vi "获取特殊单位符号字符（菜单下拉列表）.vi"(11 "特殊单位符号":T1 items=["°", "′", "″", "＄", "￥", "〒", "￠", "￡", "％", "＠", "℃", "℉", "﹩", "﹪", "‰", "﹫", "㏕", "㎜", "㎝", "㎞", "㏎", "㎡", "㎎", "㎏", "㏄", "°", "○", "¤", ""]) -> (3 "字符（双字节）":string)   [LabVIEW 2012]
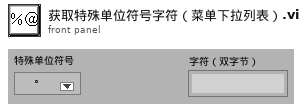
[diagram p1: front panel]
types:
  T1 = typedef "特殊单位符号菜单列表.ctl" = u16
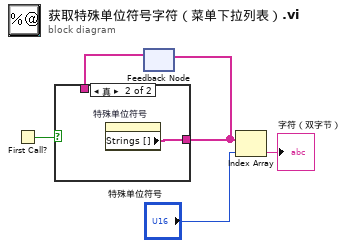
[diagram p0: block diagram]
diagram:
  n1 = First Call?() -> (First Call?: T/F=w5:bool)
  n2 = feedback #1() -> (w3:string[])  [unwired: 1 in]
  n3 = case shown="真" w5 {
    tunnel: [w6 w7] -> w4
    tunnel: w3 -> [w6 _]
    frame False {
    }
    frame True {
      n4 = property on="特殊单位符号" class="Ring (严格)"() -> ("Strings []"=w7:string[])  [unwired: 2 in, 2 out]
    }
  }
  n5 = feedback-in #1(w4) -> ()
  n6 = Index Array(array=w4, index="特殊单位符号") -> (element=→"字符（双字节）":string)
